vi "Compute 2-Exp Guess Parameters.vi"(9 "IRF":cluster{"t Array":dbl[], "Data Array":dbl[]}, 11 "Decay":cluster{"t Array":dbl[], "Data Array":dbl[]}) -> (1 "Ordered Guess Parameter Names":T1[](array[typedef])=[enum."Offset", enum."Baseline", enum."A_1", enum."tau_1", enum."A_2", enum."tau_2"], 3 "Guess Parameters":dbl[](array[numeric]))   [LabVIEW 2021, in "Fits.lvlib"]
uses:
  Fits.lvlib
  IRF(X)PSED/Decay Fit Parameters In List.ctl
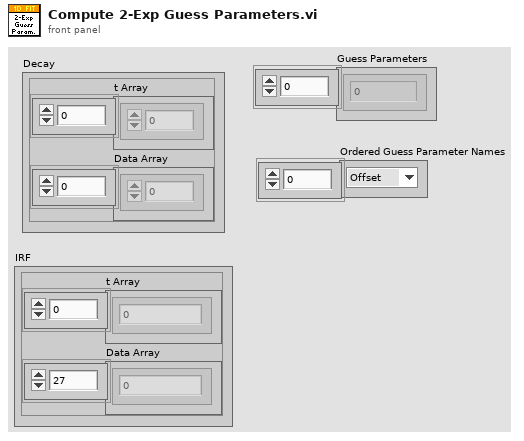
[diagram p1: front panel]
types:
  T1 = typedef "Fits.lvlib/Decay Fit Parameters In List.ctl" = enum16{"Offset", "Baseline", "A_1", "tau_1", "A_2", "tau_2"}
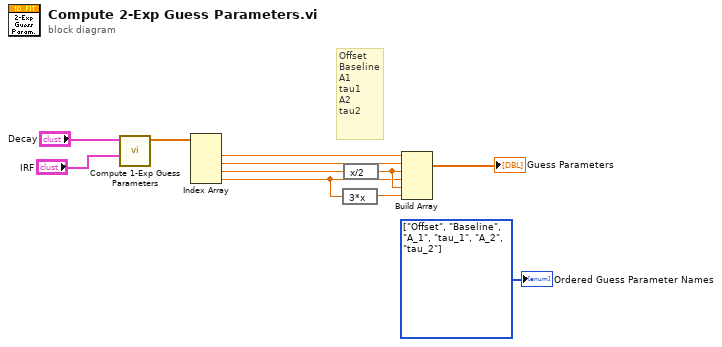
[diagram p0: block diagram]
diagram:
  w4 = T1[] [enum."Offset", enum."Baseline", enum."A_1", enum."tau_1", enum."A_2", enum."tau_2"] items=["Offset", "Baseline", "A_1", "tau_1", "A_2", "tau_2"] ("data")
  # "Offset\nBaseline\nA1\ntau1\nA2\ntau2"
  n1 = call "Compute 1-Exp Guess Parameters.vi"("IRF"="IRF", "Decay"="Decay") -> ("Guess Parameters"=w11:dbl[])  [unwired: 8 in, 1 out]
  n2 = Index Array(array=w11) -> (element #1=w6:dbl, element #2=w7:dbl, element #3=w8:dbl, element #4=w2:dbl)  [unwired: 4 in]
  n3 = expression code="3*x"(w2) -> (w3:dbl)
  n4 = expression code="x/2"(w8) -> (w9:dbl)
  n5 = Build Array(w6, w7, w9, w2, w9, w3) -> (→"Guess Parameters":dbl[])
  "Ordered Guess Parameter Names" <- w4
